vi "LM Single Exponential and gradient.vi"(3 "output control":T1, 4 "data":variant, 5 "X":dbl[](array[numeric]), 6 "a":dbl[](array[numeric])) -> (0 "error out":errorcluster, 1 "f'(X,a)":dbl[][](array[numeric]), 2 "f(X,a)":dbl[](array[numeric]))   [LabVIEW 2021, in "Fits.lvlib"]
doc: "This template is the starting point for creating a model function to be passed to the Nonlinear Curve Fit.vi."
uses:
  <vilib>/gmath/NumericalOptimization/LM_output select.ctl
  Fits.lvlib
  <vilib>/gmath/NI_Gmath.lvlib
panel:
  # "Parameters:\n\nA, t, B"
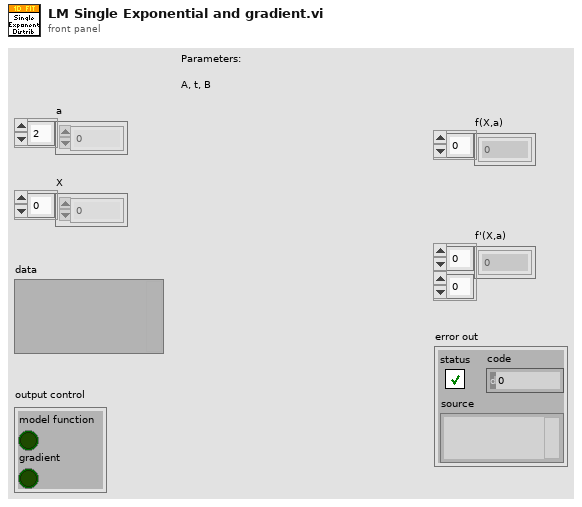
[diagram p1: front panel]
types:
  T1 = typedef "NI_Gmath.lvlib/LM_output select.ctl" = cluster{"model function":bool, "gradient":bool}
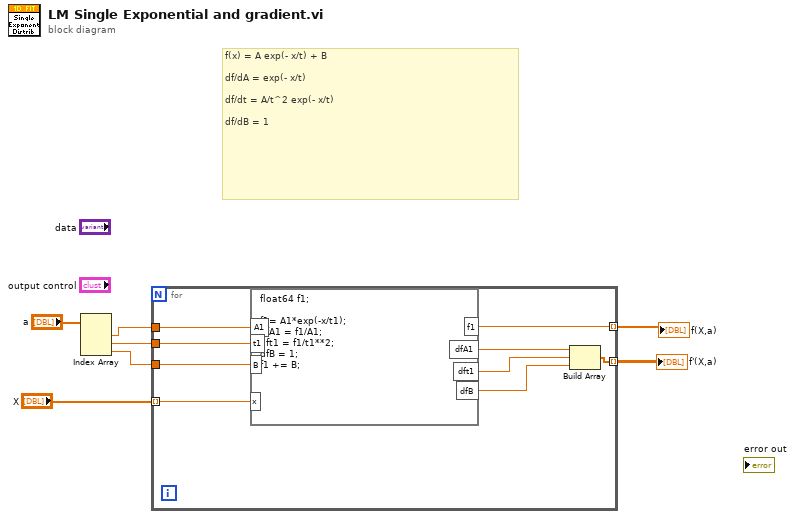
[diagram p0: block diagram]
diagram:
  # "f(x) = A exp(- x/t) + B\n\ndf/dA = exp(- x/t)     \n\ndf/dt = A/t^2 exp(- x/t) \n\ndf/dB = 1"
  n1 = Index Array(array="a") -> (element #1=w6:dbl, element #2=w5:dbl, element #3=w1:dbl)  [unwired: 3 in]
  n2 = for {
    tunnel: w6 -> [w16]
    tunnel: w5 -> [w15]
    tunnel: "X" -> [w14] mode=indexing
    tunnel: [w12] -> w3 mode=indexing
    tunnel: [w10] -> w2 mode=indexing
    tunnel: w1 -> [w9]
    n3 = formula code="float64 f1;\n\nf1= A1*exp(-x/t1);\ndfA1 = f1/A1;\ndft1 = f1/t1**2;\ndfB = 1;\nf1 += B;"("A1"=w16, "t1"=w15, "x"=w14, "B"=w9) -> ("f1"=w12:dbl, "dfA1"=w13:dbl, "dft1"=w11:dbl, "dfB"=w8:dbl)
    n4 = Build Array(w13, w11, w8) -> (w10:dbl[])
  }
  "f(X,a)" <- w3
  "f'(X,a)" <- w2
